vi "Main.vi"(11 "Module Admin":refnum<class "Delacor_lib_QMH_Module Admin.lvclass">) -> ()   [LabVIEW 2025, in "ZE_Recorder.lvlib"]
doc: "This template is based off of the Queued Message Handler design pattern and the Queued Message Handler project template that ships with LabVIEW.\n\nThe main difference is that the queue is private to this module and communication between modules is performed via Broadcast and Request events.\n\nRequest events are wrapped in public API methods and are handled in the Event Handling Loop (EHL) of this VI. Any module can register for Broadcast events sent by this module. The EHL generates messages based on user interface actions.\n\nThe Message Handling Loop (MHL) processes messages generated by the EHL, or by other messages. The messages are string values, so new messages can be added easily to the Message Cases case structure in the MHL. Each message cluster can also provide an optional value for Message Data, which is a variant that can be converted to whatever message-specific data is required.\n_____\nBased on Delacor QMH Project Template 5.0.0.82."
uses:
  ZE_Recorder.lvlib
  <vilib>/Delacor/Delacor QMH/Libraries/Module Admin_class/Delacor_lib_QMH_Module Admin.lvclass
  SaveAs.ctl
  Open.ctl
  Settings.ctl
  Start.ctl
  Stop.ctl
  Help.ctl
  Record.ctl
  ZE_Recorder_Settings.ctl
  ZE_Recorder_Header.ctl
  ZE_Recorder_ChannelCluster.ctl
  ChannelCluster.ctl
  ZE_Recorder_Units.ctl
  Temperature.ctl
  ZE_Recorder_FileCluster.ctl
  Viewer.ctl
  Module Data--cluster.ctl
  <vilib>/Delacor/Delacor QMH/Libraries/Message Queue_class/Delacor_lib_QMH_Message Queue.lvclass/Delacor_lib_QMH_Message Queue.ctl
  GuiState.ctl
  Stop Argument--cluster.ctl
  <vilib>/Delacor/Delacor QMH/Libraries/Module Admin_class/Delacor_lib_QMH_Module Admin.lvclass/Delacor_lib_QMH_Module Admin.ctl
  XmlFileAction.ctl
  ZE_Recorder_TempChannelAction.ctl
  ZE_Recorder_XMLCluster.ctl
  LVLIBP/ZE_APP_Application.lvlibp/ZE_APP_DefaultAppPaths_State.ctl
  <vilib>/Delacor/Delacor QMH/Libraries/Message Queue_class/Delacor_lib_QMH_Enqueue Message (Single).vi
  <vilib>/Delacor/Delacor QMH/Libraries/Module Admin_class/Delacor_lib_QMH_Get External Launch.vi
  <vilib>/Utility/file.llb/Write Delimited Spreadsheet (DBL).vi
  <vilib>/Utility/error.llb/Error Cluster From Error Code.vi
  <vilib>/ErrorRing/Error Ring.xnode
  <vilib>/Delacor/Delacor QMH/Libraries/Message Queue_class/Delacor_lib_QMH_Message Queue.lvclass
  LVLIBP/ZE_APP_Application.lvlibp
panel:
  in  "ReadConfig":T1
  in  "SaveConfig":T2
  out "error out":errorcluster
  out "Status":string
  in  "Settings":T3={"Header Cluster"={"Project"="", "Operator ID"="", "Description"="Measurement Description: "}, "Sampling Rate [Hz]"=100.0, "Channel Array"=[], "File Cluster"={"File Postfix"="", "Folder"=path "C:/Users/pats/Documents/LabVIEW Data", "File Type"=enum."CSV"}} caption="Header Cluster" {"Channel Array"."Terminal" items=["Default"=-1, "RSE"=10083, "NRSE"=10078, "Differential"=10106, "Pseudodifferential"=12529]; "Sampling Rate [Hz]" min=0.001 max=1000000.0 step=0.1}
  out "Title":string="ZE Recorder 4.0"
  in  "TDMSViewer":T10
  in  "Recording":T11
  in  "Help":T12
  in  "ACQ Stop":T13
  in  "ACQ Start":T14 caption="ACQ Run"
  in  "ShowSettings":T15 caption="Show Graph"
  out "Data Chart":dbl[][](graph)
  out "File":string
  out "Samples written":i64 caption="Samples\nwritten"
  # "Project Info"
  # "Channel Settings"
  # "Result File Settings"
  # "."
  # "by Zühlke SQUARE-Team"
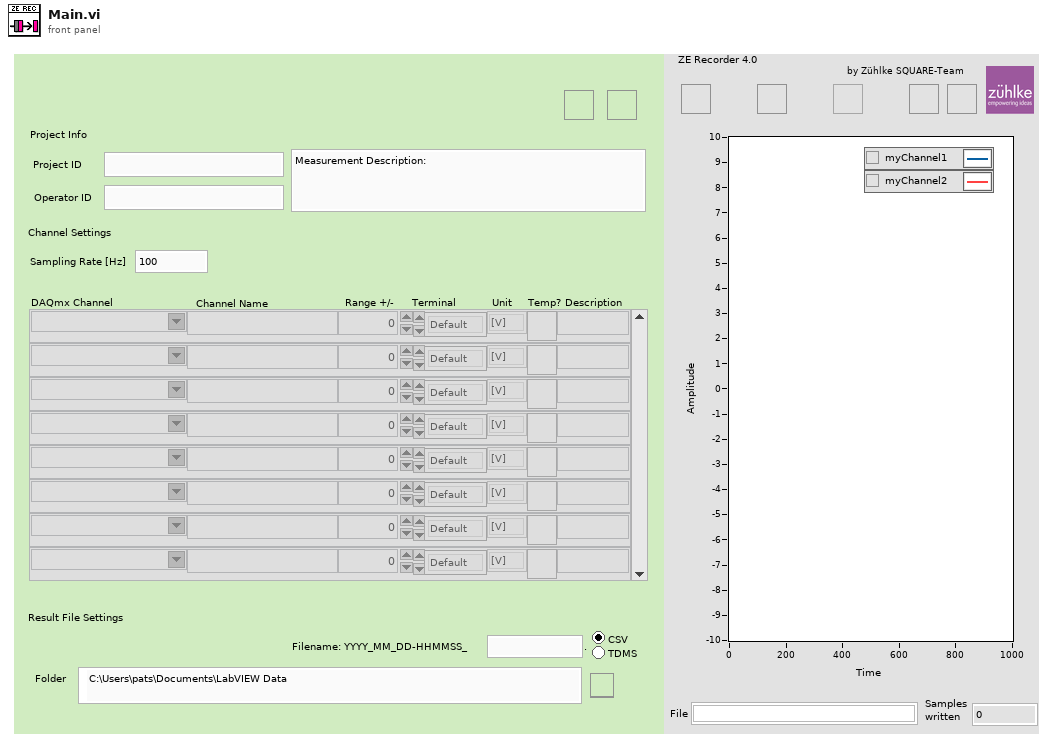
[diagram p1: front panel]
types:
  T1 = typedef "ZE_Recorder.lvlib/Open.ctl" = bool
  T2 = typedef "ZE_Recorder.lvlib/SaveAs.ctl" = bool
  T3 = typedef "ZE_Recorder.lvlib/ZE_Recorder_Settings.ctl" = cluster{"Header Cluster":T4, "Sampling Rate [Hz]":dbl, "Channel Array":T5, "File Cluster":T9}
  T4 = typedef "ZE_Recorder.lvlib/ZE_Recorder_Header.ctl" = cluster{"Project":string, "Operator ID":string, "Description":string}
  T5 = typedef "ZE_Recorder.lvlib/ZE_Recorder_ChannelCluster.ctl" = T6[]
  T6 = typedef "ZE_Recorder.lvlib/ChannelCluster.ctl" = cluster{"physical channel":tag, "channel name":string, "Range":dbl, "Terminal":i32, "Unit":T7, "isTemp":T8, "Description":string}
  T7 = typedef "ZE_Recorder.lvlib/ZE_Recorder_Units.ctl" = enum16{"[V]", "[A]", "[F]", "[H]", "[°C]", "[ml/s]", "[m/s]", "[bar]", "[%]", "[N]", "[?]"}
  T8 = typedef "ZE_Recorder.lvlib/Temperature.ctl" = bool
  T9 = typedef "ZE_Recorder.lvlib/ZE_Recorder_FileCluster.ctl" = cluster{"File Postfix":string, "Folder":path, "File Type":enum32{"CSV", "TDMS"}}
  T10 = typedef "ZE_Recorder.lvlib/Viewer.ctl" = bool
  T11 = typedef "ZE_Recorder.lvlib/Record.ctl" = bool
  T12 = typedef "ZE_Recorder.lvlib/Help.ctl" = bool
  T13 = typedef "ZE_Recorder.lvlib/Stop.ctl" = bool
  T14 = typedef "ZE_Recorder.lvlib/Start.ctl" = bool
  T15 = typedef "ZE_Recorder.lvlib/Settings.ctl" = bool
  T16 = typedef "ZE_Recorder.lvlib/Request Events--cluster.ctl" = cluster{"Stop Module":refnum<user-event>, "Show Panel":refnum<user-event>, "Hide Panel":refnum<user-event>, "Get Module Execution Status":refnum<user-event>, "Show Diagram":refnum<user-event>}
  T17 = typedef "ZE_Recorder.lvlib/Module Data--cluster.ctl" = cluster{"Status":string, "is recording?":bool, "multi Device":bool, "No of channels":i16, "ACK Tasks":refnum<k21>[], "TDMS channel array":string[], "CSV refnum":refnum<file>, "tdms refnum":refnum<k34>, "No of samples written":i64, "max Range":dbl}
  T18 = typedef "ZE_Recorder.lvlib/GuiState.ctl" = enum16{"Idle", "Acquiring"}
  T19 = enum32{"invalid lock state", "Not Locked", "Locked (No Password)", "Password-protected"}
  T20 = typedef "ZE_Recorder.lvlib/Stop Argument--cluster.ctl" = cluster{"Origin":string, "Exit via Stop Module Req?":bool, "Wait for Module to stop?":bool}
  T21 = enum32{"Invalid", "Standard", "Closed", "Hidden", "Minimized", "Maximized"}
  T22 = typedef "ZE_APP_Application.lvlibp/ZE_APP_DefaultAppPaths_State.ctl" = enum16{"Init", "Read", "Write"}
  T23 = typedef "ZE_Recorder.lvlib/ZE_Recorder_XMLCluster.ctl" = cluster{"SettingsCluster":T3}
  T24 = typedef "ZE_Recorder.lvlib/ZE_Recorder_TempChannelAction.ctl" = enum16{"Get Channel Configs", "Read Config", "Add Config", "Clear"}
  T25 = typedef "ZE_Recorder.lvlib/XmlFileAction.ctl" = enum16{"Write and Close File", "WriteFileAs", "Open File", "OpenFileWithDialog"}
  T26 = enum16{"open", "replace", "create", "open or create", "replace or create", "replace or create with confirmation"}
  T27 = enum8{"Enabled", "Disabled", "Disabled and Grayed Out"}
  T28 = typedef "LVDateTimeRec.ctl" = cluster{"fractional second":dbl, "second":i32, "minute":i32, "hour":i32, "day of month":i32, "month":i32, "year":i32, "day of week":i32, "day of year":i32, "DST":i32}
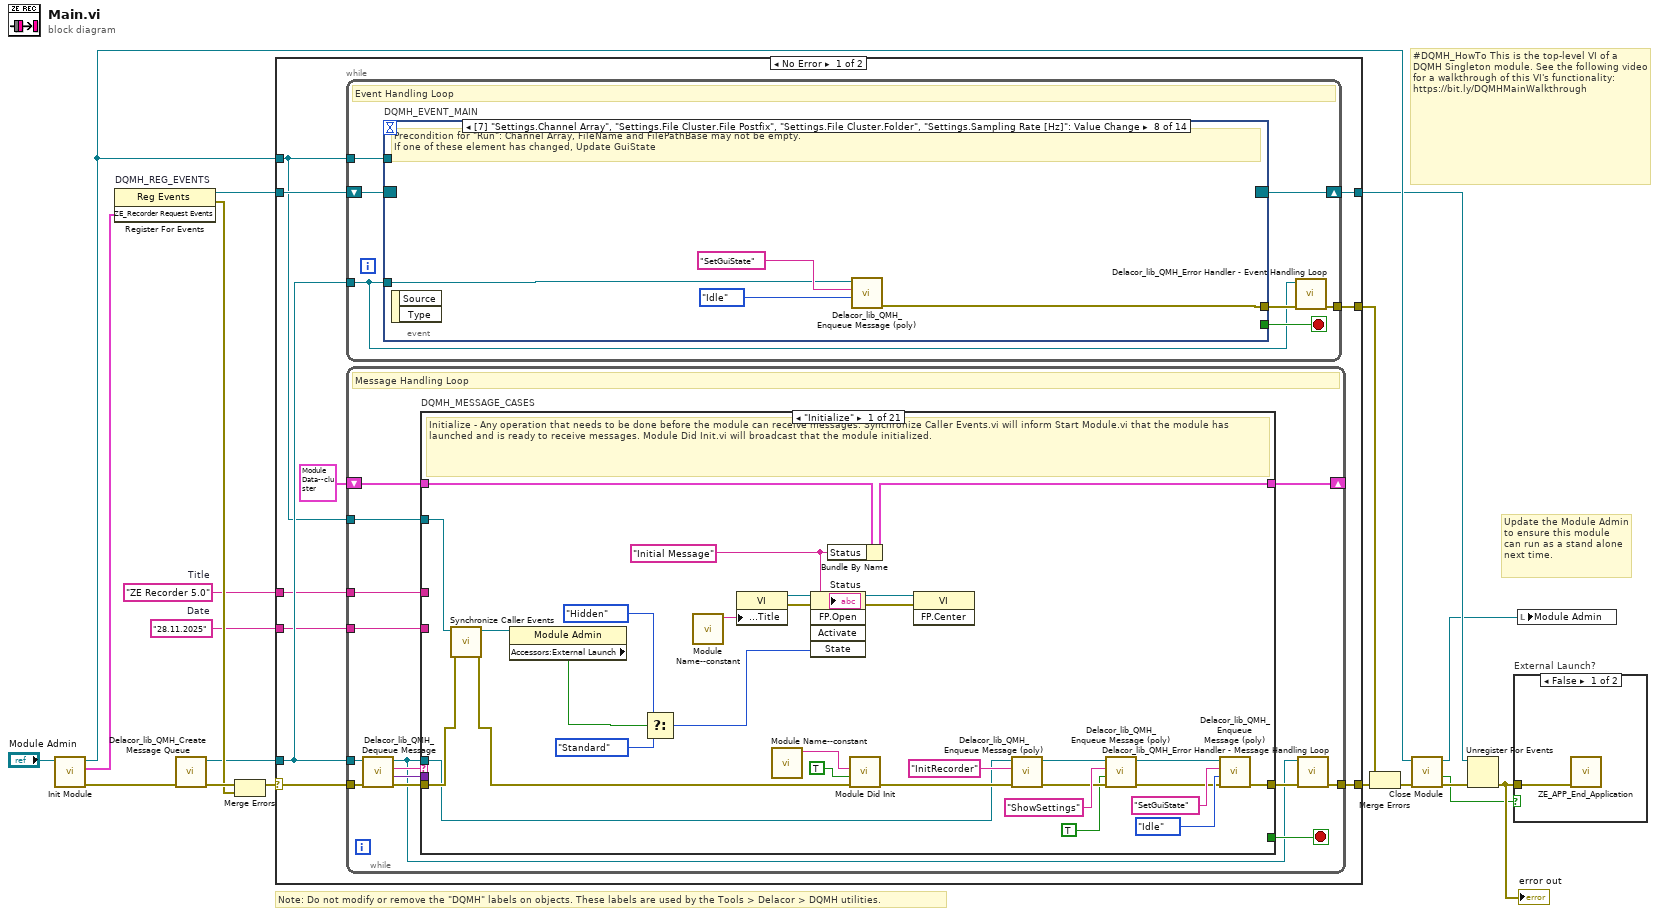
[diagram p0: block diagram]
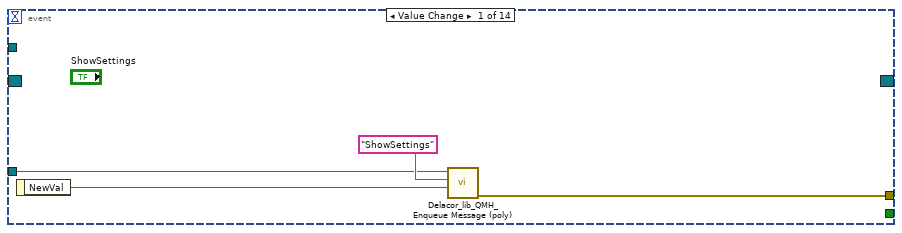
[diagram p2: hidden frame]
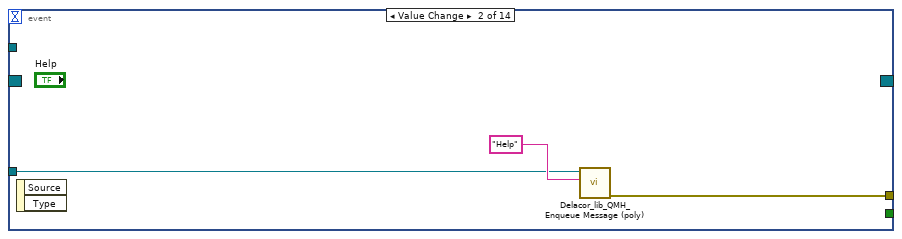
[diagram p3: hidden frame]
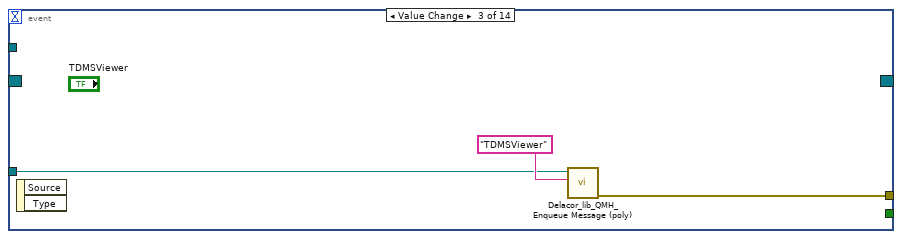
[diagram p4: hidden frame]
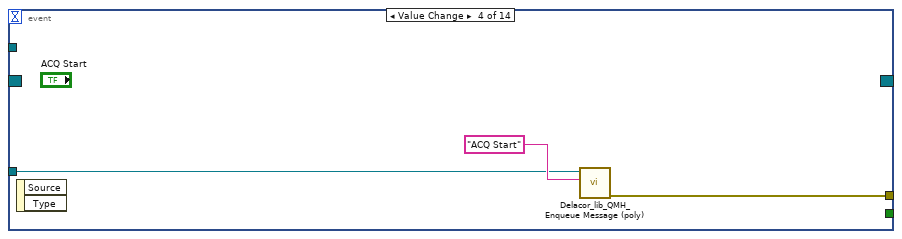
[diagram p5: hidden frame]
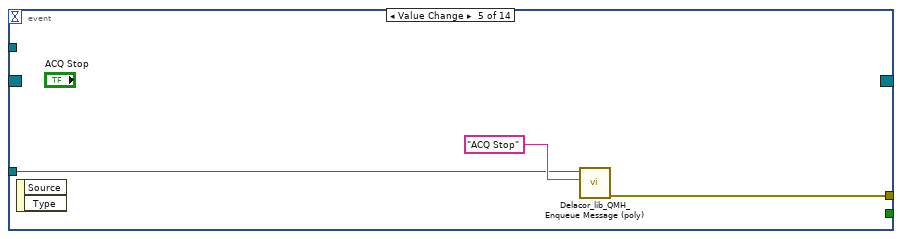
[diagram p6: hidden frame]
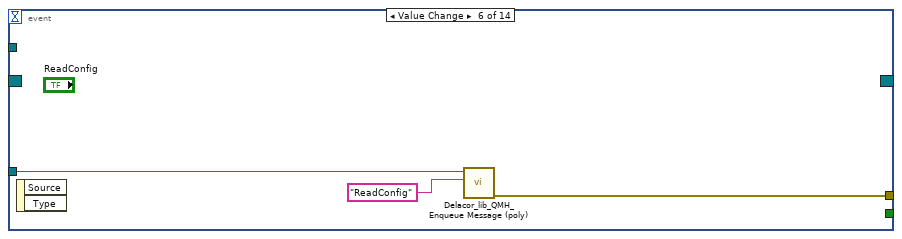
[diagram p7: hidden frame]
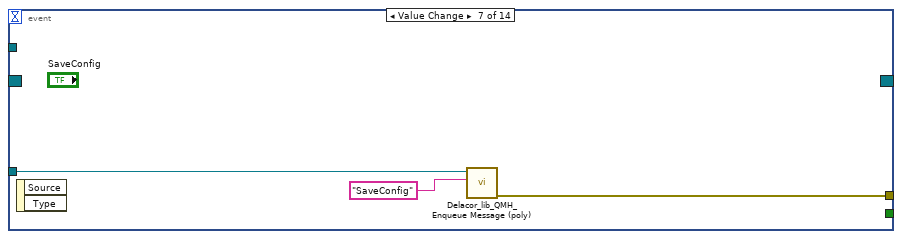
[diagram p8: hidden frame]
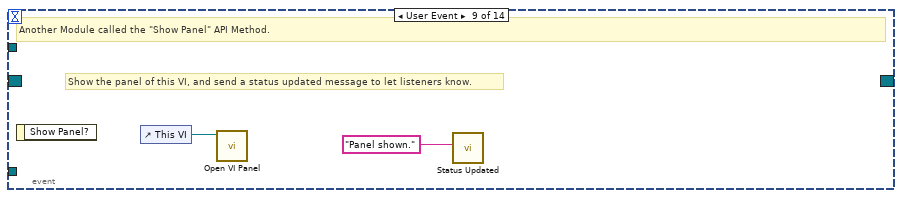
[diagram p9: hidden frame]
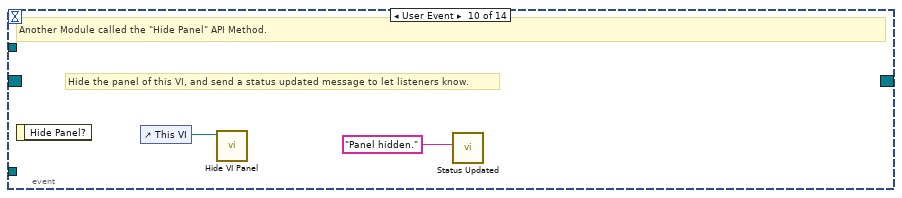
[diagram p10: hidden frame]
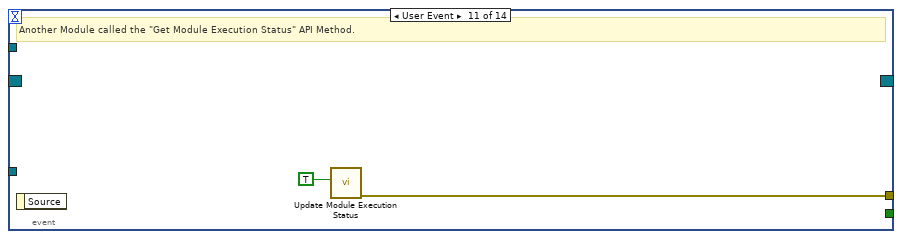
[diagram p11: hidden frame]
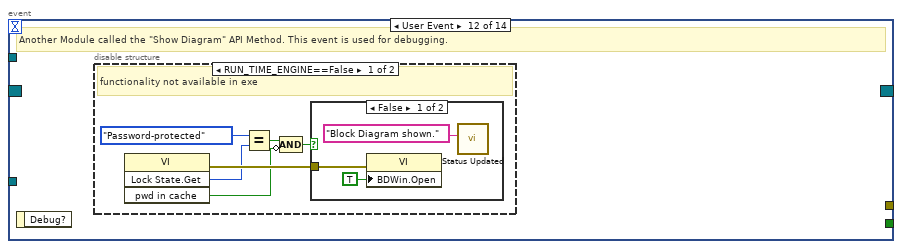
[diagram p12: hidden frame]
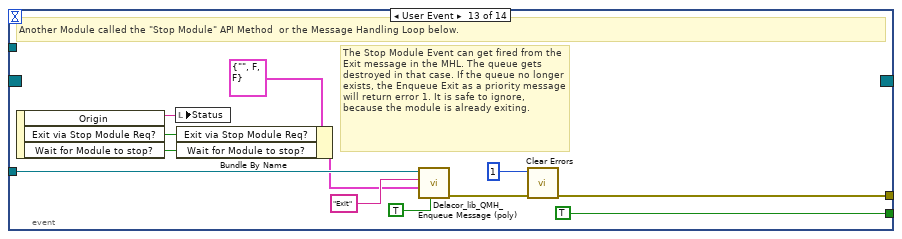
[diagram p15: hidden frame]
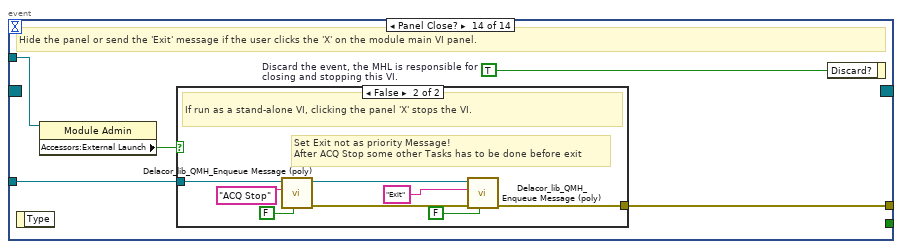
[diagram p16: hidden frame]
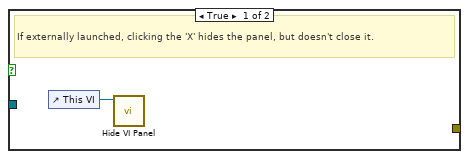
[diagram p17: hidden frame]
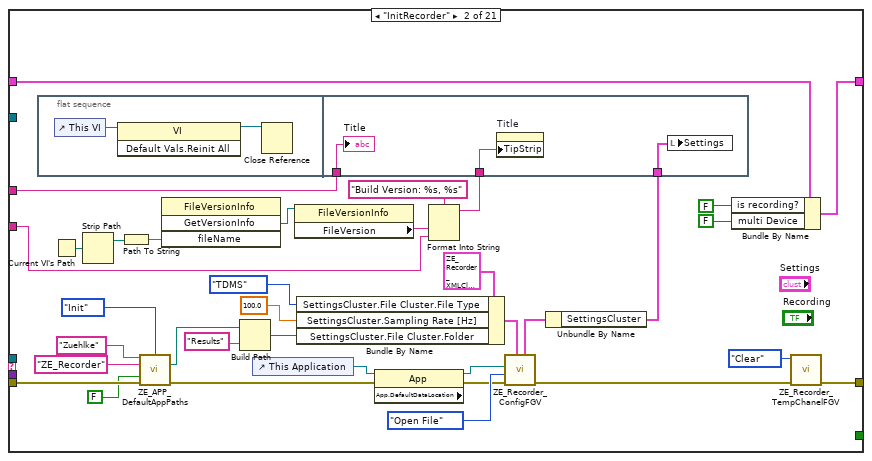
[diagram p18: hidden frame]
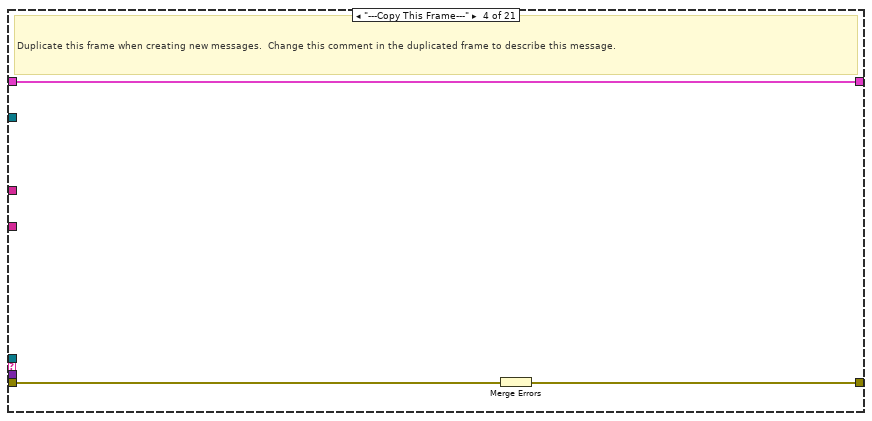
[diagram p20: hidden frame]
diagram:
  w1 = "28.11.2025"  # Date
  w2 = "ZE Recorder 5.0"  # Title
  # "#DQMH_HowTo This is the top-level VI of a DQMH Singleton module. See the following video for a walkthrough of this VI's functionality: https://bit.ly/DQMHMainWalkthrough"
  # "Note: Do not modify or remove the \"DQMH\" labels on objects. These labels are used by the Tools > Delacor > DQMH utilities."
  # "Update the Module Admin to ensure this module can run as a stand alone next time."
  n1 = call "Init Module.vi"("Singleton Module Admin in"="Module Admin") -> ("error out"=w18:errorcluster, "ZE_Recorder Request Events"=w7:T16, "Singleton Module Admin out"=w10:refnum<class "Delacor_lib_QMH_Module Admin.lvclass">)  [unwired: 8 in]
  n2 = register-events "DQMH_REG_EVENTS"(w7) -> (reference out=w8:refnum<event-registration>, error out=w11:errorcluster)  [unwired: 2 in]
  n3 = call <vilib>:"Delacor_lib_QMH_Create Message Queue.vi"("error in"=w18) -> ("error out"=w13:errorcluster, "Message Queue"=w6:refnum<class "Delacor_lib_QMH_Message Queue.lvclass">)  [unwired: 9 in]
  n4 = Merge Errors(w13, w11) -> (w12:errorcluster)
  n5 = case shown="No Error" w12 {
    selector: w12 -> [w27 w650]
    tunnel: [w29 w649] -> w19
    tunnel: [w26 w655] -> w9
    tunnel: w8 -> [w24 w655]
    tunnel: w6 -> [w23 w648]
    tunnel: [w28 _] -> w16
    tunnel: w10 -> [w22 w651]
    tunnel: w2 -> [w21 _]
    tunnel: w1 -> [w20 _]
    frame No Error {
      n6 = while {
        tunnel: w23 -> [w30]
        shift-right: [w33] -> w26
        shift-left: w24 -> [w34]
        tunnel: [w35] -> w28
        tunnel: w22 -> [w31]
        stop <- w32 stop-if-true
        # "Event Handling Loop"
        n7 = event "DQMH_EVENT_MAIN" shown="[7] \"Settings.Channel Array\", \"Settings.File Cluster.File Postfix\", \"Settings.File Cluster.Folder\", \"Settings.Sampling Rate [Hz]\": Value Change" {
          selector: w34 -> [_ _ _ _ _ _ _ _ _ _ _ _ _ _]
          dyn-events: [_ _ _ _ _ _ _ _ _ _ _ _ _ _] -> w33
          timeout: _ -> [_ _ _ _ _ _ _ _ _ _ _ _ _ _]
          tunnel: [_ _ _ _ _ _ _ _ _ _ _ _ TRUE ("Discard?") _] -> w32
          tunnel: w30 -> [w39 w41 w45 w47 w50 w54 w57 w60 _ _ _ _ w85 w92]
          tunnel: [w38 w42 w44 w48 w51 w53 w56 w59 _ _ w68 _ w88 w94] -> w36
          tunnel: w31 -> [_ _ _ _ _ _ _ _ _ _ _ _ _ w91]
          event Value Change {
            n8 = event-data() -> ("NewVal"=w37:T15)  [unwired: 1 in]
            n9 = call-poly <vilib>:"Delacor_lib_QMH_Enqueue Message (poly).vi"("Message Data"=w37, "Message"="ShowSettings", "Message Queue in"=w39) -> ("error out"=w38:errorcluster)  [unwired: 7 in, 1 out]
          }
          event Value Change {
            n10 = event-data() -> ()  [unwired: 1 in, 2 out]
            n11 = call-poly <vilib>:"Delacor_lib_QMH_Enqueue Message (poly).vi"("Message"="Help", "Message Queue in"=w41) -> ("error out"=w42:errorcluster)  [unwired: 8 in, 1 out]
          }
          event Value Change {
            n12 = event-data() -> ()  [unwired: 1 in, 2 out]
            n13 = call-poly <vilib>:"Delacor_lib_QMH_Enqueue Message (poly).vi"("Message"="TDMSViewer", "Message Queue in"=w45) -> ("error out"=w44:errorcluster)  [unwired: 8 in, 1 out]
          }
          event Value Change {
            n14 = event-data() -> ()  [unwired: 1 in, 2 out]
            n15 = call-poly <vilib>:"Delacor_lib_QMH_Enqueue Message (poly).vi"("Message"="ACQ Start", "Message Queue in"=w47) -> ("error out"=w48:errorcluster)  [unwired: 8 in, 1 out]
          }
          event Value Change {
            n16 = event-data() -> ()  [unwired: 1 in, 2 out]
            n17 = call-poly <vilib>:"Delacor_lib_QMH_Enqueue Message (poly).vi"("Message"="ACQ Stop", "Message Queue in"=w50) -> ("error out"=w51:errorcluster)  [unwired: 8 in, 1 out]
          }
          event Value Change {
            n18 = event-data() -> ()  [unwired: 1 in, 2 out]
            n19 = call-poly <vilib>:"Delacor_lib_QMH_Enqueue Message (poly).vi"("Message"="ReadConfig", "Message Queue in"=w54) -> ("error out"=w53:errorcluster)  [unwired: 8 in, 1 out]
          }
          event Value Change {
            n20 = event-data() -> ()  [unwired: 1 in, 2 out]
            n21 = call-poly <vilib>:"Delacor_lib_QMH_Enqueue Message (poly).vi"("Message"="SaveConfig", "Message Queue in"=w57) -> ("error out"=w56:errorcluster)  [unwired: 8 in, 1 out]
          }
          event Value Change {
            # "Precondition for \"Run\": Channel Array, FileName and FilePathBase may not be empty.\nIf one of these element has changed, Update GuiState"
            n22 = event-data() -> ()  [unwired: 1 in, 2 out]
            n23 = call-poly <vilib>:"Delacor_lib_QMH_Enqueue Message (poly).vi"("Message Data"=GuiState."Idle", "Message"="SetGuiState", "Message Queue in"=w60) -> ("error out"=w59:errorcluster)  [unwired: 7 in, 1 out]
          }
          event User Event {
            # "Show the panel of this VI, and send a status updated message to let listeners know."
            # "Another Module called the \"Show Panel\" API Method."
            n24 = event-data() -> ()  [unwired: 1 in, 1 out]
            n25 = control-ref of="This VI"() -> (w64:refnum<vi>)
            n26 = call "Open VI Panel.vi"("VI"=w64) -> ()  [unwired: 10 in, 1 out]
            n27 = call "Status Updated.vi"("Status"="Panel shown." ("format string")) -> ()  [unwired: 10 in, 1 out]
          }
          event User Event {
            # "Hide the panel of this VI, and send a status updated message to let listeners know."
            # "Another Module called the \"Hide Panel\" API Method."
            n28 = event-data() -> ()  [unwired: 1 in, 1 out]
            n29 = control-ref of="This VI"() -> (w66:refnum<vi>)
            n30 = call "Hide VI Panel.vi"("VI"=w66) -> ()  [unwired: 10 in, 1 out]
            n31 = call "Status Updated.vi"("Status"="Panel hidden." ("format string")) -> ()  [unwired: 10 in, 1 out]
          }
          event User Event {
            # "Another Module called the \"Get Module Execution Status\" API Method."
            n32 = event-data() -> ()  [unwired: 1 in, 1 out]
            n33 = call "Update Module Execution Status.vi"("Running?"=TRUE) -> ("error out"=w68:errorcluster)  [unwired: 10 in]
          }
          event User Event {
            # "Another Module called the \"Show Diagram\" API Method. This event is used for debugging."
            n34 = event-data() -> ()  [unwired: 1 in, 1 out]
            n35 = disable-structure shown="RUN_TIME_ENGINE==False" {
              frame condition #0 (active) {
                # "functionality not available in exe"
                n36 = invoke class="VI" method="Lock State.Get"() -> (error out=w74:errorcluster, "Get Lock State"=w73:T19, "pwd in cache"=w70:bool)  [unwired: 4 in, 1 out]
                n37 = Equal?(x=T19."Password-protected", y=w73) -> (x = y?=w71:bool)
                n38 = Compound Arithmetic op=AND(w71, invert w70) -> (w69:bool)
                n39 = case shown="False" w69 {
                  tunnel: w74 -> [w77 _]
                  frame False {
                    n40 = property class="VI"(error in=w77, "BDWin.Open"=TRUE ("Block Diagram Window:Open")) -> ()  [unwired: 1 in, 2 out]
                    n41 = call "Status Updated.vi"("Status"="Block Diagram shown." ("format string")) -> ()  [unwired: 10 in, 1 out]
                  }
                  frame True {
                    # "Password-protected VI, and the password is not in the cache. Do not show the diagram."
                  }
                }
              }
              frame condition #1 {
              }
            }
          }
          event User Event {
            # "The Stop Module Event can get fired from the Exit message in the MHL. The queue gets destroyed in that case. If the queue no longer exists, the Enqueue Exit as a priority message will return error 1. It is safe to ignore, because the module is already exiting."
            # "Another Module called the \"Stop Module\" API Method  or the Message Handling Loop below."
            n42 = event-data() -> ("Origin"=w84:string, "Exit via Stop Module Req?"=w80:bool, "Wait for Module to stop?"=w79:bool)  [unwired: 1 in]
            n43 = local write "Status"(w84) -> ()
            n44 = Bundle By Name(cluster=T20 {"Origin"="", "Exit via Stop Module Req?"=FALSE, "Wait for Module to stop?"=FALSE} ("Stop Argument"), "Exit via Stop Module Req?"=w80, "Wait for Module to stop?"=w79) -> (w78:T20)
            n45 = call-poly <vilib>:"Delacor_lib_QMH_Enqueue Message (poly).vi"("Priority Message? (F)"=TRUE, "Message Data"=w78, "Message"="Exit", "Message Queue in"=w85) -> ("error out"=w89:errorcluster)  [unwired: 6 in, 1 out]
            n46 = call <vilib>:"Clear Errors.vi"("error in (no error)"=w89, "specific error code to clear (0: all)"=1) -> ("error out"=w88:errorcluster)  [unwired: 4 in, 1 out]
          }
          event Panel Close? {
            w93 = TRUE  # Discard the event, the MHL is responsible for closing and stopping this VI.
            # "Hide the panel or send the 'Exit' message if the user clicks the 'X' on the module main VI panel."
            n47 = event-data() -> ()  [unwired: 1 in, 1 out]
            n48 = property class="Module Admin"(reference=w91) -> ("Accessors:External Launch"=w90:bool)  [unwired: 1 in, 2 out]
            n49 = case shown="False" w90 {
              tunnel: w92 -> [_ w96]
              tunnel: [_ w103] -> w94
              frame True {
                # "If externally launched, clicking the 'X' hides the panel, but doesn't close it."
                n50 = control-ref of="This VI"() -> (w95:refnum<vi>)
                n51 = call "Hide VI Panel.vi"("VI"=w95) -> ()  [unwired: 10 in, 1 out]
              }
              frame False {
                # "Set Exit not as priority Message!\nAfter ACQ Stop some other Tasks has to be done before exit"
                # "If run as a stand-alone VI, clicking the panel 'X' stops the VI."
                n52 = call-poly <vilib>:"Delacor_lib_QMH_Enqueue Message (poly).vi"("Priority Message? (F)"=FALSE, "Message"="ACQ Stop", "Message Queue in"=w96) -> ("error out"=w98:errorcluster, "Message Queue out"=w97:refnum<class "Delacor_lib_QMH_Message Queue.lvclass">)  [unwired: 7 in]
                n53 = call-poly <vilib>:"Delacor_lib_QMH_Enqueue Message (poly).vi"("Priority Message? (F)"=FALSE, "error in"=w98, "Message"="Exit", "Message Queue in"=w97) -> ("error out"=w103:errorcluster)  [unwired: 6 in, 1 out]
              }
            }
            n54 = event-data("Discard?"=w93) -> ()  [unwired: 1 in, 1 out]
          }
        }
        n55 = call-dynamic "Delacor_lib_QMH_Error Handler - Event Handling Loop.vi"("error in"=w36, "Message Queue in"=w30) -> ("dup error in"=w35:errorcluster)  [unwired: 8 in, 1 out]
      }
      n56 = while {
        tunnel: w23 -> [w108]
        shift-right: [w112] -> _
        shift-left: T17 {"Status"="", "is recording?"=FALSE, "multi Device"=FALSE, "No of channels"=0, "ACK Tasks"=[], "TDMS channel array"=[], "CSV refnum"=refnum, "tdms refnum"=refnum, "No of samples written"=0, "max Range"=0.0} ("Data Cluster") -> [w113]
        tunnel: w27 -> [w116]
        tunnel: [w114] -> w29
        tunnel: w22 -> [w106]
        tunnel: w21 -> [w105]
        tunnel: w20 -> [w104]
        stop <- w111 stop-if-true
        # "Message Handling Loop"
        n57 = call-dynamic "Delacor_lib_QMH_Dequeue Message.vi"("error in"=w116, "Message Queue in"=w108) -> ("error out"=w115:errorcluster, "Message Data"=w109:variant, "Message"=w110:string, "Message Queue out"=w107:refnum<class "Delacor_lib_QMH_Message Queue.lvclass">)  [unwired: 6 in]
        n58 = case "DQMH_MESSAGE_CASES" shown="\"Initialize\"" w110 {
          selector: w110 -> [_ _ _ _ _ _ _ _ _ _ _ _ _ _ _ _ _ _ _ _ w635]
          tunnel: w107 -> [w127 _ _ _ _ _ _ _ w276 w289 w350 w415 w475 w484 w519 _ _ _ w593 w628 _]
          tunnel: w115 -> [w145 w169 w189 w192 w194 w219 w227 w242 w272 w301 w340 w407 w476 w491 w516 w537 w544 w558 w599 w633 w637]
          tunnel: [w125 w173 w189 w191 w194 w195 w232 w245 w277 w288 w349 w416 w474 w483 w518 w538 w545 w554 w589 w616 w638] -> w117
          tunnel: w113 -> [w135 w180 w188 w190 w193 w218 w240 w246 w274 w299 w351 w405 w478 w492 w510 w536 w547 w559 w595 w615 w636]
          tunnel: [w134 w181 w188 w190 w193 w218 w240 w246 w282 w300 w352 w406 w479 w493 w511 w536 w547 w559 w595 w615 w636] -> w112
          tunnel: [_ _ _ _ _ _ _ _ _ _ _ _ _ _ _ _ _ _ _ w627 _] -> w111
          tunnel: w109 -> [_ _ _ _ _ w213 _ _ _ _ _ _ _ _ _ _ _ w557 w594 w626 _]
          tunnel: w106 -> [w136 _ _ _ _ _ _ _ _ _ _ _ _ _ _ _ _ _ w592 w621 _]
          tunnel: w105 -> [_ w160 _ _ _ _ _ _ _ _ _ _ _ _ _ _ _ _ _ _ _]
          tunnel: w104 -> [_ w151 _ _ _ _ _ _ _ _ _ _ _ _ _ _ _ _ _ _ _]
          frame "Initialize" {
            w130 = "Initial Message" ("Initial Message")
            # "Initialize - Any operation that needs to be done before the module can receive messages. Synchronize Caller Events.vi will inform Start Module.vi that the module has launched and is ready to receive messages. Module Did Init.vi will broadcast that the module initialized."
            n59 = call "Synchronize Caller Events.vi"("error in (no error)"=w145, "Singleton Module Admin in"=w136) -> ("error out"=w144:errorcluster, "Singleton Module Admin out"=w131:refnum<class "Delacor_lib_QMH_Module Admin.lvclass">)  [unwired: 8 in]
            n60 = property class="Module Admin"(reference=w131) -> ("Accessors:External Launch"=w140:bool)  [unwired: 1 in, 2 out]
            n61 = Select(t=T21."Hidden" ("State"), s=w140, f=T21."Standard" ("State")) -> (s? t:f=w137:T21)
            n62 = call "Module Name--constant.vi"() -> ("Module Name"=w143:string)  [unwired: 11 in]
            n63 = property class="VI"("Front Panel.Title"=w143) -> (reference out=w142:refnum<vi>, error out=w147:errorcluster)  [unwired: 2 in]
            n64 = call "Module Name--constant.vi"() -> ("Module Name"=w132:string)  [unwired: 11 in]
            n65 = invoke class="VI" method="FP.Open"(reference=w142, error in=w147, "State"=w137) -> (reference out=w141:refnum<vi>, error out=w146:errorcluster)  [unwired: 2 in, 3 out]
            n66 = Bundle By Name(cluster=w135, "Status"=w130) -> (w134:T17)
            n67 = call "Module Did Init.vi"("error in (no error)"=w144, "Initialized?"=TRUE, "Origin"=w132) -> ("error out"=w128:errorcluster)  [unwired: 8 in]
            n68 = invoke class="VI" method="FP.Center"(reference=w141, error in=w146) -> ()  [unwired: 1 in, 3 out]
            n69 = call-poly <vilib>:"Delacor_lib_QMH_Enqueue Message (poly).vi"("error in"=w128, "Message"="InitRecorder", "Message Queue in"=w127) -> ("error out"=w120:errorcluster, "Message Queue out"=w122:refnum<class "Delacor_lib_QMH_Message Queue.lvclass">)  [unwired: 7 in]
            n70 = call-poly <vilib>:"Delacor_lib_QMH_Enqueue Message (poly).vi"("error in"=w120, "Message Data"=TRUE ("Initialized?"), "Message"="ShowSettings", "Message Queue in"=w122) -> ("error out"=w119:errorcluster, "Message Queue out"=w121:refnum<class "Delacor_lib_QMH_Message Queue.lvclass">)  [unwired: 6 in]
            n71 = call-poly <vilib>:"Delacor_lib_QMH_Enqueue Message (poly).vi"("error in"=w119, "Message Data"=GuiState."Idle" ("GuiState"), "Message"="SetGuiState", "Message Queue in"=w121) -> ("error out"=w125:errorcluster)  [unwired: 6 in, 1 out]
            "Status" <- w130
          }
          frame "InitRecorder" {
            n72 = flat-sequence {
              tunnel: w160 -> [w187]
              tunnel: w150 -> [w186]
              tunnel: w149 -> [w185]
              frame #0 {
                n73 = control-ref of="This VI"() -> (w184:refnum<vi>)
                n74 = invoke class="VI" method="Default Vals.Reinit All"(reference=w184) -> (reference out=w183:refnum<vi>)  [unwired: 2 in, 2 out]
                n75 = Close Reference(reference=w183) -> ()  [unwired: 1 in, 1 out]
              }
              frame #1 {
                n76 = property on="Title" class="Str"("TipStrip"=w186) -> ()  [unwired: 2 in, 2 out]
                n77 = local write "Settings"(w185) -> ()
                "Title" <- w187
              }
            }
            n78 = Current VI's Path() -> (path=w156:path)
            n79 = Strip Path(path=w156) -> (stripped path=w157:path)  [unwired: 1 out]
            n80 = Path To String(path=w157) -> (string=w155:string)
            n81 = call "ZE_APP_DefaultAppPaths.vi"("Vendor"="Zuehlke", "State"=ZE_APP_DefaultAppPaths_State."Init", "Application"="ZE_Recorder", "CheckForConfigFile"=FALSE, "ErrorIn"=w169) -> ("AppDataPath"=w162:path, "ErrorOut"=w159:errorcluster)  [unwired: 7 in, 2 out]
            n82 = invoke class="FileVersionInfo" method="GetVersionInfo"("fileName"=w155) -> ("GetVersionInfo"=w154:refnum<k24>)  [unwired: 3 in, 3 out]
            n83 = Build Path(base path=w162, name or relative path="Results") -> (appended path=w164:path)
            n84 = control-ref of="This Application"() -> (w182:refnum<vi>)
            n85 = property class="FileVersionInfo"(reference=w154) -> ("FileVersion"=w152:string)  [unwired: 1 in, 2 out]
            n86 = Bundle By Name(cluster=T23 {"SettingsCluster"={"Header Cluster"={"Project"="", "Operator ID"="", "Description"="(replace) Measurement Description (replace):"}, "Sampling Rate [Hz]"=100.0, "Channel Array"=[], "File Cluster"={"File Postfix"="", "Folder"=path "C:/Users/pats/Documents/LabVIEW Data", "File Type"=enum."CSV"}}} ("XML cluster in"), "SettingsCluster.File Cluster.File Type"=enum32{"CSV", "TDMS"}."TDMS", "SettingsCluster.Sampling Rate [Hz]"=100.0, "SettingsCluster.File Cluster.Folder"=w164) -> (w171:T23)
            n87 = property class="App" props=["App.DefaultDataLocation"](reference=w182, error in=w159) -> (reference out=w176:refnum<vi>, error out=w158:errorcluster)  [unwired: 1 out]
            n88 = Format Into String(format string="Build Version: %s, %s", w152, w151) -> (resulting string=w150:string)  [unwired: 2 in, 1 out]
            n89 = call "ZE_Recorder_ConfigFGV.vi"("XML cluster in"=w171, "error in"=w158, "Action"=XmlFileAction."Open File", "Application in"=w176) -> ("error out"=w174:errorcluster, "XML cluster out"=w170:T23)  [unwired: 6 in]
            n90 = Unbundle By Name(w170) -> ("SettingsCluster"=w149:T3)
            n91 = Bundle By Name(cluster=w180, "is recording?"=FALSE, "multi Device"=FALSE) -> (w181:T17)
            n92 = call "ZE_Recorder_TempChanelFGV.vi"("error in"=w174, "Action"=ZE_Recorder_TempChannelAction."Clear") -> ("error out"=w173:errorcluster)  [unwired: 6 in, 3 out]
          }
          frame "--- Module Specific ---" {
            # "Separator -- The following cases handle messages specific to this Module."
          }
          frame "---Copy This Frame---" {
            # "Duplicate this frame when creating new messages.  Change this comment in the duplicated frame to describe this message."
            n93 = Merge Errors(w192) -> (w191:errorcluster)
          }
          frame "--- Exit and Error Handling---" {
            # "Separator - The following cases handle errors and exit messages."
          }
          frame "ShowSettings" {
            w205 = i32[] [1, 110, 220, 330, 440, 550, 650]  # animated splitterbar positions
            # "At Startup, go direct to desired position\n(no animation)"
            # "Show or Hide Settings by shifting a splitterbar left or right"
            n94 = Variant To Data(error in=w219, type=TRUE, Variant=w213) -> (data=w206:bool, error out=w208:errorcluster)
            n95 = control-ref of="This VI"() -> (w211:refnum<vi>)
            n96 = property class="VI"(reference=w211, error in=w208) -> (reference out=w214:refnum<vi>, error out=w210:errorcluster, "Panel"=w215:refnum<vi>)
            n97 = Reverse 1D Array(array=w205) -> (reversed array=w207:i32[])
            n98 = Select(t=w205, s=w206, f=w207) -> (s? t:f=w199:i32[])
            n99 = property class="Pnl"(reference=w215, error in=w210) -> (error out=w209:errorcluster, "Splitters[]"=w204:refnum<vi>[])  [unwired: 1 out]
            n100 = Reverse 1D Array(array=w199) -> (reversed array=w202:i32[])
            n101 = Array Subset(array=w202, length=1) -> (w200:i32[])  [unwired: 1 in]
            n102 = First Call?() -> (First Call?: T/F=w203:bool)
            n103 = Index Array(array=w204, index=0) -> (element=w217:refnum<vi>)
            n104 = Select(t=w200, s=w203, f=w199) -> (s? t:f=w198:i32[])
            n105 = for {
              tunnel: w198 -> [w224] mode=indexing
              tunnel: w217 -> [w223]
              shift-right: [w221] -> w197
              shift-left: w209 -> [w222]
              n106 = property class="Splitter"(reference=w223, error in=w222, "Position"=w224) -> (error out=w221:errorcluster)  [unwired: 1 out]
              n107 = Wait (ms)(milliseconds to wait=u32 20) -> ()  [unwired: 1 out]
            }
            n108 = Close Reference(reference=w204, error in (no error)=w197) -> (error out=w196:errorcluster)
            n109 = Close Reference(reference=w214, error in (no error)=w196) -> (error out=w195:errorcluster)
          }
          frame "Help" {
            # "Open Helpfile (pdf)"
            n110 = call "ZE_APP_DefaultAppPaths.vi"("State"=ZE_APP_DefaultAppPaths_State."Read", "ErrorIn"=w227) -> ("AppDataPath"=w229:path, "ErrorOut"=w228:errorcluster)  [unwired: 10 in, 2 out]
            n111 = Build Path(base path=w229, name or relative path="Config") -> (appended path=w226:path)
            n112 = Build Path(base path=w226, name or relative path="ZE RecorderHelpFile.pdf") -> (appended path=w236:path)
            n113 = Path To String(path=w236) -> (string=w235:string)
            n114 = Concatenate Strings("cmd /c\"" ("string"), w235, "\"" ("string")) -> (w233:string)
            n115 = call <vilib>:"System Exec.vi"("run minimized? (F)"=TRUE, "wait until completion? (T)"=FALSE, "error in (no error)"=w228, "command line"=w233) -> ("error out"=w232:errorcluster)  [unwired: 4 in, 3 out]
          }
          frame "TDMSViewer" {
            w244 = FALSE  # Write
            # "Opens a TDMS Viewer Window with File Dialog. If a Measurement is running, use the actual filename as startvalue of the filedialog"
            n116 = call "TDMSViewerRunningFlag.vi"("Write"=w244, "error in"=w242) -> ("RunningOut"=w241:bool, "error out"=w243:errorcluster)  [unwired: 12 in]
            n117 = case shown="False" w241 {
              tunnel: [w252 w267] -> w245
              tunnel: w243 -> [w251 w267]
              frame False {
                w254 = 128  # call and forget
                # "If File is an empty sting,\npass folder without filename to Viewer"
                # "TDMS Viewer is not yet running, start Viewer async."
                n118 = local read "Settings"() -> (w255:T3)
                n119 = local read "File"() -> (w247:string)
                n120 = Unbundle By Name(w255) -> ("File Cluster.Folder"=w249:path)
                n121 = Current VI's Path() -> (path=w257:path)
                n122 = Strip Path(path=w257) -> (stripped path=w258:path)  [unwired: 1 out]
                n123 = Build Path(base path=w258, name or relative path="TDMSViewerStart.vi") -> (appended path=w256:path)
                n124 = case shown="\"\"" w247 {
                  selector: w247 -> [_ w264]
                  tunnel: w249 -> [w263 w266]
                  tunnel: [w263 w265] -> w248
                  frame "" {
                  }
                  frame Default {
                    n125 = Build Path(base path=w266, name or relative path=w264) -> (appended path=w265:path)
                  }
                }
                n126 = Open VI Reference(type specifier VI Refnum (for type only)=refnum<vi> refnum, vi path=w256, options=w254, error in (no error)=w251) -> (vi reference=w250:refnum<vi>, error out=w253:errorcluster)  [unwired: 2 in]
                n127 = call-by-ref "Start Asynchronous Call"(reference=w250, error in=w253, "TDMSFilePath"=w248) -> (reference out=w262:refnum<vi>, error out=w261:errorcluster)  [unwired: 15 in]
                n128 = Close Reference(reference=w262, error in (no error)=w261) -> (error out=w252:errorcluster)
              }
              frame True {
                # "TDMS Viewer is alrady running, ignore comand"
              }
            }
          }
          frame "ACQ Start" {
            n129 = local read "Settings"() -> (w273:T3)
            n130 = Unbundle By Name(w273) -> ("Channel Array"=w269:T5)
            n131 = Array Size(array=w269) -> (size(s)=w268:i32)
            n132 = call-poly <vilib>:"Delacor_lib_QMH_Enqueue Message (poly).vi"("error in"=w272, "Message Data"=GuiState."Acquiring" ("GuiState"), "Message"="SetGuiState", "Message Queue in"=w276) -> ("error out"=w278:errorcluster, "Message Queue out"=w275:refnum<class "Delacor_lib_QMH_Message Queue.lvclass">)  [unwired: 6 in]
            n133 = property on="Data Chart" class="WFChart (strict)"(error in=w272, "History Data"=dbl[][] [], "LegNumRows"=w268) -> (error out=w270:errorcluster)  [unwired: 1 in, 1 out]
            n134 = for {
              tunnel: w269 -> [w287] mode=indexing
              tunnel: w270 -> [w286]
              i -> [w285]
              n135 = Unbundle By Name(w287) -> ("channel name"=w284:string)
              n136 = property on="Data Chart" class="WFChart (strict)"(error in=w286, "Active Plot"=w285, "Plot.Plot Name"=w284) -> ()  [unwired: 1 in, 2 out]
            }
            n137 = Bundle By Name(cluster=w274, "is recording?"=TRUE ("Acquiring")) -> (w282:T17)
            n138 = call-poly <vilib>:"Delacor_lib_QMH_Enqueue Message (poly).vi"("error in"=w278, "Message"="CreateTasks", "Message Queue in"=w275) -> ("error out"=w277:errorcluster)  [unwired: 7 in, 1 out]
          }
          frame "CreateTasks" {
            # "write back reordered channels"
            n139 = local read "Settings"() -> (w293:T3)
            n140 = Unbundle By Name(w293) -> ("Channel Array"=w294:T5, "Sampling Rate [Hz]"=w290:dbl)
            n141 = call "ZE_Recorder_CheckChannelDuplicates.vi"("Channel Array"=w294) -> ("Multi Device"=w296:bool, "No of channels"=w295:i16, "Channel Array out"=w291:T5)  [unwired: 7 in, 1 out]
            n142 = case shown="1, Default" w295 {
              tunnel: w301 -> [w313 w326]
              tunnel: [w304 w329] -> w298
              tunnel: w290 -> [w310 _]
              tunnel: w291 -> [w312 _]
              tunnel: [w311 5.0 ("max Range")] -> w297
              tunnel: w296 -> [w309 _]
              tunnel: w289 -> [w307 w327]
              tunnel: [w306 w325] -> w288
              frame 1, Default {
                n143 = call "ZE_Recorder_InitializeTask.vi"("error in (no error)"=w313, "Sampling Rate [Hz]"=w310, "Multi devices?"=w309, "Channel Array in"=w312) -> ("error out"=w308:errorcluster, "Array"=w305:refnum<k21>[], "max Range"=w311:dbl)  [unwired: 5 in]
                n144 = for {
                  tunnel: w305 -> [w323] mode=indexing
                  tunnel: [w322] -> w304 mode=indexing
                  tunnel: [w321] -> w303 mode=indexing
                  n145 = call <vilib>:"DAQmx Start Task.vi"("task/channels in"=w323) -> ("task out"=w322:refnum<k21>, "error out"=w321:errorcluster)  [unwired: 13 in]
                }
                n146 = Merge Errors(w303) -> (w302:errorcluster)
                n147 = case shown="No Error" w302 {
                  selector: w302 -> [_ w319]
                  tunnel: w308 -> [w317 w320]
                  tunnel: w307 -> [w315 _]
                  tunnel: [w314 w318] -> w306
                  frame No Error {
                    n148 = call-poly <vilib>:"Delacor_lib_QMH_Enqueue Message (poly).vi"("error in"=w317, "Message"="CreateFile", "Message Queue in"=w315) -> ("error out"=w314:errorcluster)  [unwired: 7 in, 1 out]
                  }
                  frame Error {
                    n149 = Merge Errors(w320, w319) -> (w318:errorcluster)
                  }
                }
              }
              frame -1 {
                n150 = Build Array(refnum<k21> refnum ("task out")) -> (w329:refnum<k21>[])
                n151 = call-poly <vilib>:"Delacor_lib_QMH_Enqueue Message (poly).vi"("error in"=w326, "Message Data"=GuiState."Idle" ("GuiState"), "Message"="SetGuiState", "Message Queue in"=w327) -> ("error out"=w325:errorcluster)  [unwired: 6 in, 1 out]
              }
            }
            n152 = Bundle By Name(cluster=w293, "Channel Array"=w291) -> (w292:T3)
            n153 = local write "Settings"(w292) -> ()
            n154 = Bundle By Name(cluster=w299, "No of channels"=w295, "multi Device"=w296, "max Range"=w297, "ACK Tasks"=w298) -> (w300:T17)
          }
          frame "CreateFile" {
            # "Create Folder if it does not exist"
            n155 = local read "Settings"() -> (w345:T3)
            n156 = Unbundle By Name(w345) -> ("Header Cluster"=w332:T4, "Sampling Rate [Hz]"=w333:dbl, "Channel Array"=w334:T5, "File Cluster.File Type"=w347:enum32{"CSV", "TDMS"}, "File Cluster.File Postfix"=w346:string, "File Cluster.Folder"=w339:path)
            n157 = Get Date/Time In Seconds() -> (seconds since 1Jan1904=w357:timestamp)
            n158 = Seconds To Date/Time(time stamp (now)=w357) -> (date time rec=w337:T28)  [unwired: 1 in]
            n159 = call <vilib>:"Check if File or Folder Exists.vi"("error in (no error)"=w340, "path"=w339) -> ("error out"=w342:errorcluster, "file or folder exists?"=w343:bool, "dup path"=w344:path)  [unwired: 7 in]
            n160 = case shown="False" w343 {
              tunnel: w344 -> [w361 w362]
              tunnel: w342 -> [w360 w363]
              tunnel: [w359 w363] -> w341
              tunnel: [w358 w362] -> w338
              frame False {
                n161 = Create Folder(path (use dialog)=w361, error in=w360) -> (created path=w358:path, error out=w359:errorcluster)  [unwired: 1 in, 1 out]
              }
              frame True {
              }
            }
            n162 = call "ZE_Recorder_CreatePath.vi"("date time rec"=w337, "File Path Base"=w338, "File Name"=w346) -> ("file path"=w353:path)  [unwired: 7 in, 1 out]
            n163 = case shown="\"TDMS\"" w347 {
              tunnel: w353 -> [w379 w392]
              tunnel: w341 -> [w381 w395]
              tunnel: [w374 w389] -> w348
              tunnel: [refnum<k34> refnum ("tdms file out") w388] -> w354
              tunnel: [w375 refnum<file> refnum ("refnum out")] -> w355
              tunnel: [string[] [] w387] -> w356
              tunnel: [w372 w386] -> w336
              tunnel: w334 -> [_ w385]
              tunnel: w333 -> [_ w384]
              tunnel: w332 -> [_ w383]
              frame "CSV", Default {
                n164 = Path To String(path=w379) -> (string=w378:string)
                n165 = Concatenate Strings(w378, ".csv" ("name or relative path")) -> (w376:string)
                n166 = String To Path(string=w376) -> (path=w372:path)
                n167 = Open/Create/Replace File(file path (use dialog)=w372, error in=w381, operation (0:open)=T26."create") -> (refnum out=w375:refnum<file>, error out=w374:errorcluster)  [unwired: 3 in, 1 out]
              }
              frame "TDMS" {
                n168 = Path To String(path=w392) -> (string=w391:string)
                n169 = Concatenate Strings(w391, ".tdms" ("name or relative path")) -> (w393:string)
                n170 = String To Path(string=w393) -> (path=w386:path)
                n171 = call "ZE_Recorder_CreateTDMS.vi"("Header Cluster"=w383, "Sampling Rate [Hz]"=w384, "error in (no error)"=w395, "Channel Array"=w385, "TDMS Path"=w386) -> ("error out"=w389:errorcluster, "Name Array"=w387:string[], "TDMS Refnum out"=w388:refnum<k34>)  [unwired: 4 in]
              }
            }
            n172 = Strip Path(path=w336) -> (name=→"File":string)  [unwired: 1 out]
            n173 = case shown="Error" w348 {
              selector: w348 -> [w364 _]
              tunnel: w350 -> [w366 w369]
              tunnel: [w365 w368] -> w349
              frame No Error {
                n174 = call-poly <vilib>:"Delacor_lib_QMH_Enqueue Message (poly).vi"("error in"=w364, "Message"="ACQ and Write Data", "Message Queue in"=w366) -> ("error out"=w365:errorcluster)  [unwired: 7 in, 1 out]
              }
              frame Error {
                n175 = One Button Dialog(message="Problems creating File \nThe path already exists. Please  rename or try again later.") -> ()  [unwired: 1 in, 1 out]
                n176 = call-poly <vilib>:"Delacor_lib_QMH_Enqueue Message (poly).vi"("Message"="CloseTasks", "Message Queue in"=w369) -> ("error out"=w368:errorcluster)  [unwired: 8 in, 1 out]
              }
            }
            n177 = Bundle By Name(cluster=w351, "CSV refnum"=w355, "tdms refnum"=w354, "TDMS channel array"=w356) -> (w352:T17)
          }
          frame "ACQ and Write Data" {
            n178 = Unbundle By Name(w405) -> ("No of samples written"=w414:i64, "tdms refnum"=w412:refnum<k34>, "CSV refnum"=w411:refnum<file>, "TDMS channel array"=w409:string[], "ACK Tasks"=w396:refnum<k21>[], "No of channels"=w397:i16, "is recording?"=w398:bool)
            n179 = local read "Settings"() -> (w402:T3)
            n180 = Unbundle By Name(w402) -> ("File Cluster.File Type"=w401:enum32{"CSV", "TDMS"}, "Sampling Rate [Hz]"=w400:dbl)
            n181 = case shown="True" w398 {
              tunnel: [w418 w424] -> w408
              tunnel: w396 -> [_ w423]
              tunnel: w397 -> [_ w422]
              tunnel: w407 -> [w418 w421]
              tunnel: w400 -> [_ w420]
              tunnel: [dbl[][] [] ("data") w419] -> w399
              frame False {
              }
              frame True {
                n182 = call "ZE_Recorder_ReadFromTasks.vi"("error in"=w421, "sampling rate"=w420, "No of channels"=w422, "ACK Tasks"=w423) -> ("error out"=w424:errorcluster, "data"=w419:dbl[][])  [unwired: 6 in]
              }
            }
            n183 = Empty Array?(array=w399) -> (empty?=w413:bool)
            n184 = case shown="False" w413 {
              tunnel: [w435 w457] -> w403
              tunnel: w399 -> [w425 _]
              tunnel: w414 -> [w434 w457]
              tunnel: w401 -> [w433 _]
              tunnel: w412 -> [w432 _]
              tunnel: w411 -> [w431 _]
              tunnel: "Measurement Data" ("group name in (Untitled)") -> [w430 _]
              tunnel: w409 -> [w429 _]
              tunnel: w408 -> [w428 w456]
              tunnel: [w427 w456] -> w404
              frame False {
                n185 = case shown="\"TDMS\"" w433 {
                  tunnel: w428 -> [w445 w454]
                  tunnel: w432 -> [_ w453]
                  tunnel: w431 -> [w447 _]
                  tunnel: w425 -> [w443 w451]
                  tunnel: [w445 w448] -> w427
                  tunnel: w430 -> [_ w455]
                  tunnel: w429 -> [_ w452]
                  frame "CSV", Default {
                    n186 = Refnum to Path(1:w447) -> (0:w446:path)
                    n187 = Transpose 2D Array(2D array=w443) -> (transposed array=w442:dbl[][])
                    n188 = call-poly <vilib>:"Write Delimited Spreadsheet.vi"("file path (dialog if empty)"=w446, "format (%.3f)"="%.8e", "2D data"=w442, "append to file? (new file:F)"=TRUE, "transpose? (no:F)"=FALSE, "delimiter (\\t)"=";" ("delimiter (\\t)")) -> ()  [unwired: 8 in, 2 out]
                  }
                  frame "TDMS" {
                    n189 = TDMS Write(0:w453, 5:w455, 7:w452, 9:w451, 11:w454) -> (4:w450:refnum<k34>, 15:w449:errorcluster)  [unwired: 1 in, 2 out]
                    n190 = TDMS Flush(4:w449, 7:w450) -> (0:w448:errorcluster)  [unwired: 1 out]
                  }
                }
                n191 = Array Size(array=w425) -> (size(s)=w438:i32[])
                n192 = Transpose 2D Array(2D array=w425) -> (transposed array=→"Data Chart":dbl[][])
                n193 = Index Array(array=w438, index=1) -> (element=w436:i32)
                n194 = Add(x=w434, y=w436) -> (x+y=w435:i64)
              }
              frame True {
              }
            }
            "Samples written" <- w403
            n195 = case shown="True" w398 {
              tunnel: [w458 w467] -> w416
              tunnel: w404 -> [w458 w466]
              tunnel: w415 -> [_ w465]
              frame False {
              }
              frame True {
                # "blink recording"
                n196 = Tick Count (ms)() -> (millisecond timer value=w462:u32)
                n197 = feedback #1() -> (w461:u32)  [unwired: 1 in]
                n198 = Subtract(x=w462, y=w461) -> (x-y=w464:u32)
                n199 = Greater?(x=w464, y=u32 500) -> (0:w463:bool)
                n200 = case shown="True" w463 {
                  tunnel: w462 -> [_ w470]
                  tunnel: [w469 w470] -> w459
                  tunnel: w461 -> [w469 _]
                  frame False {
                  }
                  frame True {
                    n201 = property on="Recording" class="Bool (strict)"() -> ("Visible"=w472:bool)  [unwired: 2 in, 2 out]
                    n202 = Not(x=w472) -> (.not. x?=w471:bool)
                    n203 = property on="Recording" class="Bool (strict)"("Visible"=w471) -> ()  [unwired: 2 in, 2 out]
                  }
                }
                n204 = feedback-in #1(w459) -> ()
                n205 = call-poly <vilib>:"Delacor_lib_QMH_Enqueue Message (poly).vi"("error in"=w466, "Message"="ACQ and Write Data", "Message Queue in"=w465) -> ("error out"=w467:errorcluster)  [unwired: 7 in, 1 out]
              }
            }
            n206 = Bundle By Name(cluster=w405, "No of samples written"=w403) -> (w406:T17)
          }
          frame "ACQ Stop" {
            n207 = Bundle By Name(cluster=w478, "is recording?"=FALSE ("Acquiring")) -> (w479:T17)
            n208 = call-poly <vilib>:"Delacor_lib_QMH_Enqueue Message (poly).vi"("Priority Message? (F)"=TRUE, "error in"=w476, "Message"="CloseFile", "Message Queue in"=w475) -> ("error out"=w474:errorcluster)  [unwired: 6 in, 1 out]
          }
          frame "CloseFile" {
            n209 = local read "Settings"() -> (w490:T3)
            n210 = Unbundle By Name(w490) -> ("File Cluster.File Type"=w486:enum32{"CSV", "TDMS"}, "Header Cluster"=w487:T4, "Channel Array"=w488:T5, "Sampling Rate [Hz]"=w489:dbl)
            n211 = Unbundle By Name(w492) -> ("CSV refnum"=w494:refnum<file>, "tdms refnum"=w495:refnum<k34>, "No of samples written"=w496:i64)
            n212 = call "ZE_Recorder_CreateHeader.vi"("Sampling Rate"=w489, "No Samples"=w496, "Channel Array"=w488, "Header Cluster"=w487) -> ("TDMS propValues"=w502:string[], "TDMS properties"=w503:string[], "Header out"=w501:string)  [unwired: 5 in]
            n213 = call "ZE_Recorder_AddHeaderToFile.vi"("property values"=w502, "property names"=w503, "Header in"=w501, "error in"=w491, "File Type"=w486, "tdms refnum"=w495, "csv refnum in"=w494) -> ("error out"=w500:errorcluster)  [unwired: 4 in]
            n214 = flat-sequence {
              tunnel: [refnum<file> refnum ("refnum out")] -> w497
              tunnel: [refnum<k34> refnum ("tdms file out")] -> w498
              tunnel: [i16 0 ("No of samples written")] -> w499
              tunnel: w500 -> [w504]
              tunnel: [w504] -> w482
              frame #0 {
              }
            }
            n215 = Bundle By Name(cluster=w492, "No of samples written"=w499, "CSV refnum"=w497, "tdms refnum"=w498) -> (w493:T17)
            n216 = call-poly <vilib>:"Delacor_lib_QMH_Enqueue Message (poly).vi"("Priority Message? (F)"=TRUE, "error in"=w482, "Message"="CloseTasks", "Message Queue in"=w484) -> ("error out"=w483:errorcluster)  [unwired: 6 in, 1 out]
          }
          frame "CloseTasks" {
            # "Don't care about errors here"
            n217 = Unbundle By Name(w510) -> ("ACK Tasks"=w517:refnum<k21>[])
            n218 = for {
              shift-right: [w522] -> w515
              shift-left: w516 -> [w523]
              tunnel: w517 -> [w521] mode=indexing
              # "no active task?"
              n219 = Equal?(x=w521, y=refnum<k21> refnum ("ACQ task")) -> (x = y?=w524:bool)
              n220 = case shown="True" w524 {
                tunnel: w523 -> [w527 w529]
                tunnel: [w526 w529] -> w522
                tunnel: w521 -> [w528 _]
                frame False {
                  n221 = call <vilib>:"DAQmx Clear Task.vi"("task in"=w528, "error in"=w527) -> ("error out"=w526:errorcluster)  [unwired: 13 in]
                }
                frame True {
                }
              }
            }
            n222 = Build Array(refnum<k21> refnum ("ACQ task")) -> (w513:refnum<k21>[])
            n223 = call <vilib>:"Clear Errors.vi"("error in (no error)"=w515) -> ("error out"=w514:errorcluster)  [unwired: 5 in, 1 out]
            n224 = Bundle By Name(cluster=w510, "ACK Tasks"=w513) -> (w511:T17)
            n225 = call-poly <vilib>:"Delacor_lib_QMH_Enqueue Message (poly).vi"("Priority Message? (F)"=TRUE, "error in"=w514, "Message Data"=GuiState."Idle" ("GuiState"), "Message"="SetGuiState", "Message Queue in"=w519) -> ("error out"=w518:errorcluster)  [unwired: 5 in, 1 out]
          }
          frame "ReadConfig" {
            # "Read Configuration File with file dialog"
            n226 = local read "Settings"() -> (w531:T3)
            n227 = Bundle By Name(cluster=T23 {"SettingsCluster"={"Header Cluster"={"Project"="", "Operator ID"="", "Description"="(replace) Measurement Description (replace):"}, "Sampling Rate [Hz]"=100.0, "Channel Array"=[], "File Cluster"={"File Postfix"="", "Folder"=path "C:/Users/pats/Documents/LabVIEW Data", "File Type"=enum."CSV"}}} ("XML cluster in"), "SettingsCluster"=w531) -> (w533:T23)
            n228 = control-ref of="This Application"() -> (w532:refnum<vi>)
            n229 = call "ZE_Recorder_ConfigFGV.vi"("XML cluster in"=w533, "error in"=w537, "Action"=XmlFileAction."OpenFileWithDialog", "Application in"=w532) -> ("error out"=w538:errorcluster, "XML cluster out"=w535:T23)  [unwired: 6 in]
            n230 = Unbundle By Name(w535) -> ("SettingsCluster"=w530:T3)
            n231 = local write "Settings"(w530) -> ()
          }
          frame "SaveConfig" {
            # "SaveConig file with file dialog"
            n232 = local read "Settings"() -> (w541:T3)
            n233 = control-ref of="This Application"() -> (w543:refnum<vi>)
            n234 = Bundle By Name(cluster=T23 {"SettingsCluster"={"Header Cluster"={"Project"="", "Operator ID"="", "Description"="(replace) Measurement Description (replace):"}, "Sampling Rate [Hz]"=100.0, "Channel Array"=[], "File Cluster"={"File Postfix"="", "Folder"=path "C:/Users/pats/Documents/LabVIEW Data", "File Type"=enum."CSV"}}} ("XML cluster in"), "SettingsCluster"=w541) -> (w540:T23)
            n235 = call "ZE_Recorder_ConfigFGV.vi"("XML cluster in"=w540, "error in"=w544, "Action"=XmlFileAction."WriteFileAs", "Application in"=w543) -> ("error out"=w545:errorcluster)  [unwired: 6 in, 1 out]
          }
          frame "SetGuiState" {
            # "Enable or Disable GUI Elements"
            n236 = Variant To Data(error in=w558, type=GuiState."Idle", Variant=w557) -> (data=w556:T18, error out=w555:errorcluster)
            n237 = case shown="\"Idle\", Default" w556 {
              tunnel: w555 -> [w582 w588]
              tunnel: [w582 w588] -> w554
              tunnel: [w566 T27."Disabled and Grayed Out" ("Disabled")] -> w552
              tunnel: [T27."Disabled and Grayed Out" ("Disabled") T27."Enabled" ("Disabled")] -> w551
              tunnel: [T27."Enabled" ("Disabled") T27."Disabled and Grayed Out" ("Disabled")] -> w548
              tunnel: [T27."Enabled" ("Disabled") T27."Disabled and Grayed Out" ("Disabled")] -> w550
              tunnel: [T27."Enabled" ("Disabled") T27."Disabled and Grayed Out" ("Disabled")] -> w549
              frame "Idle", Default {
                # "Check if preconditions for \"Run\" are missing"
                n238 = local read "Settings"() -> (w572:T3)
                n239 = property on="Recording" class="Bool (strict)"("Value"=T11 FALSE ("Recording"), "Visible"=FALSE) -> ()  [unwired: 2 in, 2 out]
                n240 = Unbundle By Name(w572) -> ("Channel Array"=w573:T5, "File Cluster.File Postfix"=w574:string, "File Cluster.Folder"=w575:path, "Sampling Rate [Hz]"=w561:dbl)
                n241 = Empty Array?(array=w573) -> (empty?=w569:bool)
                n242 = Empty String/Path?(string/path=w574) -> (empty?=w570:bool)
                n243 = Less Or Equal To 0?(x=w561) -> (x <= 0?=w560:bool)
                n244 = Empty String/Path?(string/path=w575) -> (empty?=w571:bool)
                n245 = Compound Arithmetic op=OR(w569, w570, w571, w560) -> (w565:bool)
                n246 = Select(t="Start Acquiring\nChannel List, File Name and Folder may not be empty. Sampling Rate may not be Zero" ("Message"), s=w565, f="Start Acquiring" ("Message")) -> (s? t:f=w564:string)
                n247 = property on="ACQ Start" class="Bool"("TipStrip"=w564) -> ()  [unwired: 2 in, 2 out]
                n248 = Select(t=T27."Disabled and Grayed Out" ("Disabled"), s=w565, f=T27."Enabled" ("Disabled")) -> (s? t:f=w566:T27)
              }
              frame "Acquiring" {
              }
            }
            n249 = property on="ACQ Start" class="Bool"("DisabledEnum"=w552) -> ()  [unwired: 2 in, 2 out]
            n250 = property on="ACQ Stop" class="Bool"("DisabledEnum"=w551) -> ()  [unwired: 2 in, 2 out]
            n251 = property on="ReadConfig" class="Bool"("DisabledEnum"=w550) -> ()  [unwired: 2 in, 2 out]
            n252 = property on="SaveConfig" class="Bool"("DisabledEnum"=w549) -> ()  [unwired: 2 in, 2 out]
            n253 = property on="Channel Array" class="Arr (strict)"("DisabledEnum"=w548) -> ()  [unwired: 2 in, 2 out]
            n254 = property on="Sampling Rate [Hz]" class="DigNum (strict)"("DisabledEnum"=w548) -> ()  [unwired: 2 in, 2 out]
            n255 = property on="File Cluster" class="Clust (strict)"("DisabledEnum"=w548) -> ()  [unwired: 2 in, 2 out]
            n256 = disable-structure shown="Disabled" {
              frame Disabled {
                n257 = property on="Settings" class="Clust (strict)" props=["DisabledEnum"]() -> ()  [unwired: 3 in, 2 out]
              }
              frame Enabled {
              }
            }
          }
          frame "Error" {
            # "#CodeRecommended - If the module is running in standalone mode (External Launch = FALSE), this code will pop up an error dialog and call the 'Exit' message if an error occurs. Add more fine-grained error handling here."
            # "Error - Check the error message data and respond accordingly. This message is sent by the \"Error Handler\" VIs at the end of each loop in this application."
            n258 = property class="Module Admin"(reference=w592) -> ("Accessors:External Launch"=w591:bool)  [unwired: 1 in, 2 out]
            n259 = Variant To Data(error in=w599, type=errorcluster {"status"=FALSE, "code"=0, "source"=""} ("error constant"), Variant=w594) -> (data=w600:errorcluster, error out=w597:errorcluster)
            n260 = call "Module Name--constant.vi"() -> ("Module Name"=w590:string)  [unwired: 11 in]
            n261 = call "Error Reported.vi"("Additional Information"=w590, "Error"=w600) -> ()  [unwired: 9 in, 1 out]
            n262 = case shown="False" w591 {
              tunnel: [w603 _] -> w596
              tunnel: w593 -> [w601 _]
              tunnel: w600 -> [w602 _]
              frame False {
                # "If the module is running standalone, then pop up an error dialog and call the \"Exit\" message."
                n263 = disable-structure shown="Enabled" {
                  disable-tunnel: [w607 w608] -> w603
                  disable-tunnel: w601 -> [w606 w609]
                  frame Disabled {
                    n264 = call-poly <vilib>:"Delacor_lib_QMH_Enqueue Message (poly).vi"("Priority Message? (F)"=TRUE, "Message"="Exit", "Message Queue in"=w606) -> ("error out"=w607:errorcluster)  [unwired: 7 in, 1 out]
                  }
                  frame Enabled {
                    n265 = call-poly <vilib>:"Delacor_lib_QMH_Enqueue Message (poly).vi"("Priority Message? (F)"=FALSE, "Message"="ACQ Stop", "Message Queue in"=w609) -> ("error out"=w608:errorcluster)  [unwired: 7 in, 1 out]
                  }
                }
                n266 = call <vilib>:"Simple Error Handler.vi"("error in (no error)"=w602) -> ()  [unwired: 4 in, 5 out]
              }
              frame True {
                # "If the module was launched externally, calling the Error Reported broadcast VI is the only action performed by the \"Error\" message. The module's caller can then process the error appropriately."
              }
            }
            n267 = Merge Errors(w597, w596) -> (w589:errorcluster)
            n268 = local write "error out"(w589) -> ()
          }
          frame "Exit" {
            w625 = 91  # 91: not all Exit messages will have an argument
            w627 = TRUE  # Stop the VI
            # "Release the message queue reference"
            # "Exit - Exit the application."
            n269 = Variant To Data(error in=w633, type=T20 {"Origin"="", "Exit via Stop Module Req?"=FALSE, "Wait for Module to stop?"=FALSE} ("Stop Argument"), Variant=w626) -> (data=w623:T20, error out=w630:errorcluster)
            n270 = call <vilib>:"Clear Errors.vi"("error in (no error)"=w630, "specific error code to clear (0: all)"=w625) -> ("error out"=w632:errorcluster)  [unwired: 4 in, 1 out]
            n271 = control-ref of="This VI"() -> (w622:refnum<vi>)
            n272 = call-dynamic "Delacor_lib_QMH_Release Message Queue.vi"("error in"=w632, "Message Queue"=w628) -> ("error out"=w631:errorcluster)  [unwired: 9 in]
            n273 = call "Handle Exit.vi"("Stop Argument"=w623, "Admin in"=w621, "VI reference"=w622) -> ("error out"=w629:errorcluster)  [unwired: 7 in, 1 out]
            n274 = Merge Errors(w631, w629) -> (w617:errorcluster)
            n275 = local read "Settings"() -> (w612:T3)
            n276 = control-ref of="This Application"() -> (w619:refnum<vi>)
            n277 = Bundle By Name(cluster=T23 {"SettingsCluster"={"Header Cluster"={"Project"="", "Operator ID"="", "Description"="(replace) Measurement Description (replace):"}, "Sampling Rate [Hz]"=100.0, "Channel Array"=[], "File Cluster"={"File Postfix"="", "Folder"=path "C:/Users/pats/Documents/LabVIEW Data", "File Type"=enum."CSV"}}} ("XML cluster in"), "SettingsCluster"=w612) -> (w614:T23)
            n278 = call "ZE_Recorder_ConfigFGV.vi"("XML cluster in"=w614, "error in"=w617, "Action"=XmlFileAction."Write and Close File", "Application in"=w619) -> ("error out"=w620:errorcluster)  [unwired: 6 in, 1 out]
            n279 = Close Reference(reference=w619, error in (no error)=w620) -> (error out=w616:errorcluster)
          }
          frame Default {
            # "'Default' case only runs if there is a message that isn't defined in any of the other cases.  Output a programming error."
            n280 = call "Module Name--constant.vi"() -> ("Module Name"=w634:string)  [unwired: 11 in]
            n281 = xnode "Error Ring"("parameter 0"=w635, "parameter 1"=w634) -> ("error out"=w639:errorcluster)
            n282 = Merge Errors(w637, w639) -> (w638:errorcluster)
          }
        }
        n283 = call-dynamic "Delacor_lib_QMH_Error Handler - Message Handling Loop.vi"("error in"=w117, "Message Queue in"=w107) -> ("dup error in"=w114:errorcluster)  [unwired: 8 in, 1 out]
      }
    }
    frame Error {
      # "Synchronize Caller Events.vi will inform Start Module.vi that the module has launched and will let the code calling Start Module.vi register for broadcasts and would permit the caller receive the broadcast that an error occurred at launch time."
      n284 = call-dynamic "Delacor_lib_QMH_Release Message Queue.vi"("error in"=w650, "Message Queue"=w648) -> ("error out"=w649:errorcluster)  [unwired: 9 in]
      n285 = call "Synchronize Caller Events.vi"("Singleton Module Admin in"=w651) -> ("error out"=w656:errorcluster)  [unwired: 9 in, 1 out]
      n286 = call "Module Name--constant.vi"() -> ("Module Name"=w654:string)  [unwired: 11 in]
      n287 = Format Into String(format string="An error occurred during initialization. %s is no longer running.", w654) -> (resulting string=w652:string)  [unwired: 2 in, 1 out]
      n288 = Merge Errors(w649, w656) -> (w657:errorcluster)
      n289 = call "Error Reported.vi"("Additional Information"=w652, "Error"=w657) -> ()  [unwired: 9 in, 1 out]
    }
  }
  n290 = Merge Errors(w16, w19) -> (w15:errorcluster)
  n291 = call "Close Module.vi"("error in (no error)"=w15, "Module Admin in"=w10) -> ("error out"=w17:errorcluster, "External Launch"=w3:bool, "Module Admin out"=w4:refnum<class "Delacor_lib_QMH_Module Admin.lvclass">)  [unwired: 7 in]
  n292 = Unregister For Events(event registration refnum=w9, error in=w17) -> (error out=w14:errorcluster)
  "error out" <- w14
  n293 = case "External Launch?" shown="False" w3 {
    tunnel: w14 -> [w658 w659]
    frame False {
      n294 = call "ZE_APP_End_Application.vi"("ErrorIn"=w658) -> ()  [unwired: 15 in]
    }
    frame True {
      n295 = case shown="No Error" w659 {
        frame No Error {
          n296 = invoke class="VI" method="FP.Close"() -> ()  [unwired: 3 in, 3 out]
        }
        frame Error {
          n297 = invoke class="VI" method="FP.Open"("Activate"=TRUE ("Activate?")) -> ()  [unwired: 4 in, 5 out]
        }
      }
    }
  }
  n298 = local write "Module Admin"(w4) -> ()
